vi "List.vi"(7 "Qualified Name":string, 8 "error in (no error)":errorcluster, 11 "ConfigManager in":refnum<class "ConfigManager.lvclass">) -> (0 "error out":errorcluster, 2 "Keys":string[](array[string]), 3 "ConfigManager out":refnum<class "ConfigManager.lvclass">)   [LabVIEW 2013, in "CfgManager.lvlib" / "ConfigManager.lvclass"]
uses:
  ConfigManager.lvclass
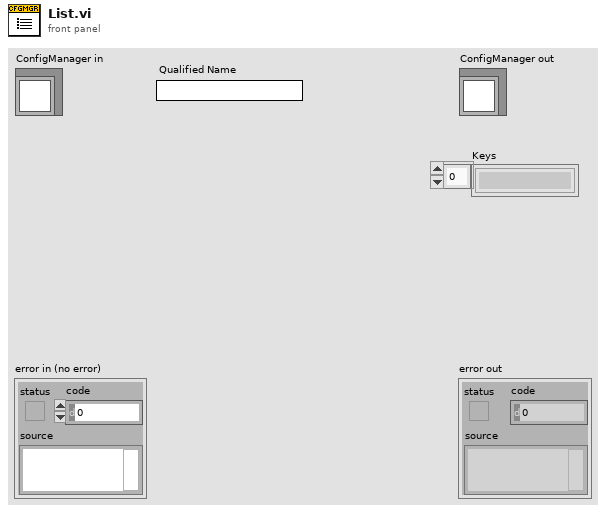
[diagram p1: front panel]
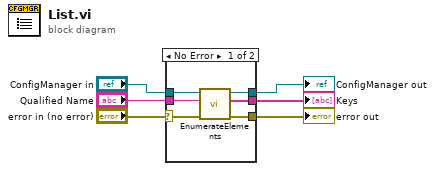
[diagram p0: block diagram]
diagram:
  n1 = case shown="No Error" "error in (no error)" {
    selector: "error in (no error)" -> [w7 w13]
    tunnel: "Qualified Name" -> [w12 _]
    tunnel: [w11 _] -> w5
    tunnel: "ConfigManager in" -> [w10 w14]
    tunnel: [w9 w14] -> w3
    tunnel: [w8 w13] -> w2
    frame No Error {
      n2 = call-dynamic "EnumerateElements.vi"("error in (no error)"=w7, "Qualified Name"=w12, "ConfigManager in"=w10) -> ("error out"=w8:errorcluster, "keys"=w11:string[], "ConfigManager out"=w9:refnum<class "ConfigManager.lvclass">)  [unwired: 6 in]
    }
    frame Error {
    }
  }
  "error out" <- w2
  "ConfigManager out" <- w3
  "Keys" <- w5
